vi "writeToXML.vi"(8 "error in (no error)":errorcluster, 10 "Class Label":string="Elevation", 11 "Elevation in":refnum<class "Elevation.lvclass">) -> (0 "error out":errorcluster, 2 "XML out":string="<>\n  <degreesAlt>90</degreesAlt>\n  <minutesArc>0</minutesArc>\n  <secondsArc>0</secondsArc>\n</>", 3 "Elevation out":refnum<class "Elevation.lvclass">)   [LabVIEW 2014, in "TCSDataDefinitions.lvlib" / "TCSCommand.lvlib" / "TargetConfiguration.lvlib" / "Target.lvlib" / "FixedTarget.lvlib" / "Elevation.lvclass"]
uses:
  Elevation.lvclass
  <userlib>/Common/UnitsAndXML/FlattenItemWithUnitToXML/FlattenPlaneAngleToXML/PlaneAngleUnit.ctl
  Elevation.lvclass/Elevation.ctl
  <userlib>/Common/UnitsAndXML/UnitsAndXML.lvlib
  <userlib>/Common/XML/XMLGenerator/XMLGenerator.lvclass
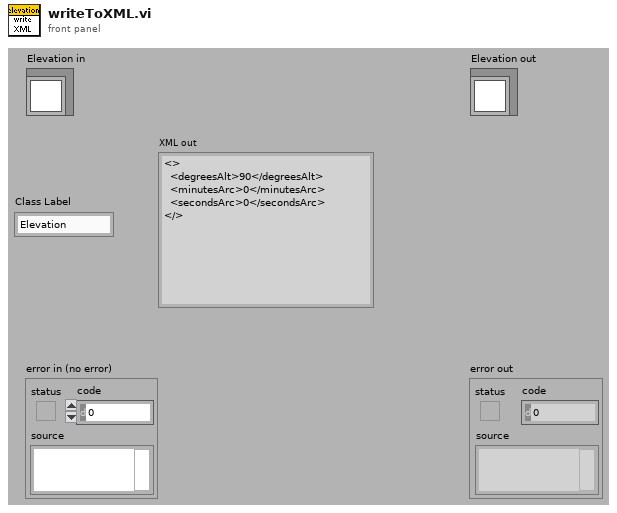
[diagram p1: front panel]
types:
  T1 = typedef "UnitsAndXML.lvlib/PlaneAngleUnit.ctl" = enum16{"rad", "deg", "'", "\""}
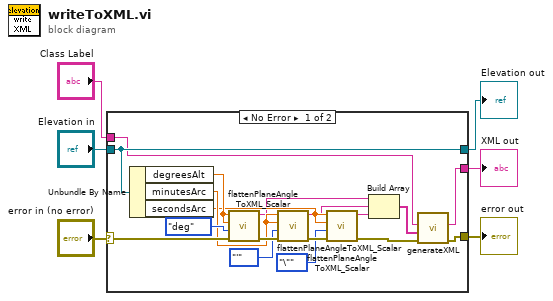
[diagram p0: block diagram]
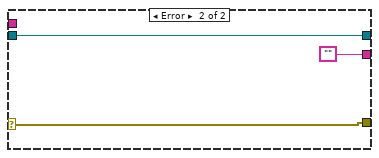
[diagram p2: hidden frame]
diagram:
  n1 = case shown="No Error" "error in (no error)" {
    selector: "error in (no error)" -> [w21 w27]
    tunnel: [w8 w27] -> w5
    tunnel: [w10 w26] -> w3
    tunnel: "Elevation in" -> [w10 w26]
    tunnel: [w9 ""] -> w2
    tunnel: "Class Label" -> [w7 _]
    frame No Error {
      n2 = Unbundle By Name(w10) -> ("degreesAlt"=w22:dbl[unit], "minutesArc"=w17:dbl[unit], "secondsArc"=w16:dbl[unit])
      n3 = call <userlib>:"flattenPlaneAngleToXML_Scalar.vi"("error in (no error)"=w21, "planeAngleUnitInXML"=PlaneAngleUnit."deg", "planeAngleAgain"=w22, "planeAngle"=w22) -> ("error out"=w24:errorcluster, "xmlString"=w15:string)  [unwired: 6 in]
      n4 = call <userlib>:"flattenPlaneAngleToXML_Scalar.vi"("error in (no error)"=w24, "planeAngleUnitInXML"=PlaneAngleUnit."'", "planeAngleAgain"=w17, "planeAngle"=w17) -> ("error out"=w23:errorcluster, "xmlString"=w14:string)  [unwired: 6 in]
      n5 = call <userlib>:"flattenPlaneAngleToXML_Scalar.vi"("error in (no error)"=w23, "planeAngleUnitInXML"=PlaneAngleUnit."\"", "planeAngleAgain"=w16, "planeAngle"=w16) -> ("error out"=w12:errorcluster, "xmlString"=w13:string)  [unwired: 6 in]
      n6 = Build Array(w15, w14, w13) -> (w11:string[])
      n7 = call <userlib>:"generateXML.vi"("error in"=w12, "childrenXML"=w11, "elementName"=w7) -> ("error out"=w8:errorcluster, "XML out"=w9:string)  [unwired: 6 in, 1 out]
    }
    frame Error {
    }
  }
  "error out" <- w5
  "Elevation out" <- w3
  "XML out" <- w2
